vi "Blend.vi"(7 "Source Name in":string, 8 "error in (no error)":errorcluster, 9 "Source Enqueuer":refnum<class "Message Enqueuer.lvclass">, 10 "Sample to Blend in":refnum<class "Sample.lvclass">, 11 "Preparation Line in":refnum<class "Preparation Line.lvclass">) -> (0 "error out":errorcluster, 2 "Source Name":string, 3 "Preparation Line out":refnum<class "Preparation Line.lvclass">)   [LabVIEW 2015, in "cRIO-Carbondioxide.lvlib" / "CO2-Actor.lvlib" / "Preparation Line.lvclass"]
uses:
  Preparation Line.lvclass
  subs/Sample/Sample.lvclass
  <vilib>/ActorFramework/Message Enqueuer/Message Enqueuer.lvclass
  Valve/Valve.lvclass
  Preparation Line.lvclass/Preparation Line.ctl
  CO2 Actor Messages/Ping Msg/Ping Msg.lvclass/Ping Msg.ctl
  <vilib>/ActorFramework/Message Enqueuer/Message Enqueuer.lvclass/Message Enqueuer.ctl
  <vilib>/ActorFramework/Message Enqueuer/Enqueue.vi
  <vilib>/ActorFramework/Message Priority Queue/Priority Enqueue.vi
  CO2 Actor/CO2 Actor.lvclass
  CO2 Actor Messages/Ping Msg/Ping Msg.lvclass
  <vilib>/ActorFramework/Actor/Actor.lvclass
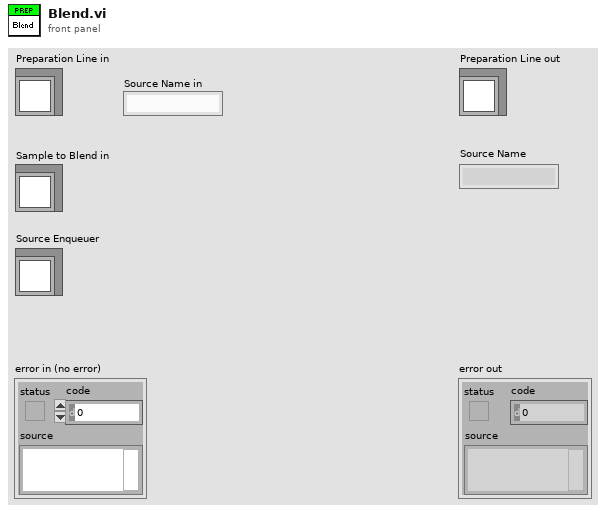
[diagram p1: front panel]
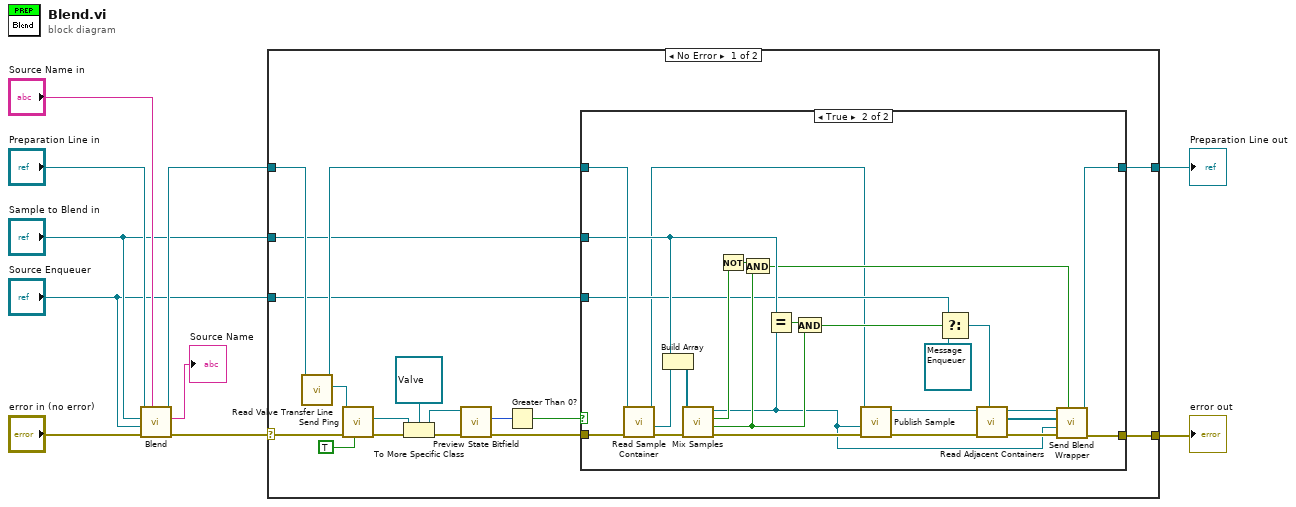
[diagram p0: block diagram]
diagram:
  n1 = call-parent "Blend.vi"("Source Name in"="Source Name in", "error in (no error)"="error in (no error)", "Source Enqueuer"="Source Enqueuer", "Sample to Blend in"="Sample to Blend in", "CO2 Actor in"="Preparation Line in") -> ("error out"=w4:errorcluster, "Source Name"=→"Source Name":string, "CO2 Actor out"=w6:refnum<class "Preparation Line.lvclass">)  [unwired: 4 in]
  n2 = case shown="No Error" w4 {
    selector: w4 -> [w26 w56]
    tunnel: w6 -> [w27 w55]
    tunnel: [w14 w55] -> w5
    tunnel: "Sample to Blend in" -> [w16 _]
    tunnel: "Source Enqueuer" -> [w15 _]
    tunnel: [w13 w56] -> w1
    frame No Error {
      n3 = call "Read Valve Transfer Line.vi"("Preparation Line in"=w27) -> ("Actor Framework:Message Enqueuer"=w25:refnum<class "Message Enqueuer.lvclass">, "Preparation Line out"=w17:refnum<class "Preparation Line.lvclass">)  [unwired: 9 in]
      n4 = call "Send Ping.vi"("Return Self (F)"=TRUE, "error in (no error)"=w26, "Message Enqueuer"=w25) -> ("error out"=w24:errorcluster, "Actor out"=w23:refnum<class "Actor.lvclass">)  [unwired: 5 in, 2 out]
      n5 = To More Specific Class(target class=refnum<class "Valve.lvclass"> refnum ("Valve.lvclass"), reference=w23, error in=w24) -> (specific class reference=w19:refnum<class "Valve.lvclass">, error out=w21:errorcluster)
      n6 = call "Preview State Bitfield.vi"("error in (no error)"=w21, "Valve in"=w19) -> ("error out"=w20:errorcluster, "State Bitfield"=w18:u16)  [unwired: 7 in, 1 out]
      n7 = Greater Than 0?(x=w18) -> (x > 0?=w12:bool)
      n8 = case shown="True" w12 {
        tunnel: w20 -> [w28 w54]
        tunnel: w17 -> [w29 w50]
        tunnel: w16 -> [_ w48]
        tunnel: w15 -> [_ w41]
        tunnel: [w29 w32] -> w14
        tunnel: [w28 w31] -> w13
        frame False {
        }
        frame True {
          n9 = call "Read Sample Container.vi"("error in (no error)"=w54, "Preparation Line in"=w50) -> ("error out"=w53:errorcluster, "Sample"=w52:refnum<class "Sample.lvclass">, "Preparation Line out"=w33:refnum<class "Preparation Line.lvclass">)  [unwired: 6 in, 1 out]
          n10 = Build Array(w48, w52) -> (w51:refnum<class "Sample.lvclass">[])
          n11 = call "Mix Samples.vi"("error in (no error)"=w53, "Samples In"=w51) -> ("error out"=w49:errorcluster, "is clean?"=w43:bool, "Empty Samples present?"=w46:bool, "Sample out"=w30:refnum<class "Sample.lvclass">)  [unwired: 6 in]
          n12 = Not(x=w46) -> (.not. x?=w47:bool)
          n13 = And(x=w47, y=w43) -> (x .and. y?=w45:bool)
          n14 = Equal?(x=w48, y=w30) -> (x = y?=w44:bool)
          n15 = And(x=w44, y=w43) -> (x .and. y?=w42:bool)
          n16 = call "Publish Sample.vi"("error in (no error)"=w49, "Sample"=w30, "Preparation Line in"=w33) -> ("error out"=w38:errorcluster, "Preparation Line out"=w37:refnum<class "Preparation Line.lvclass">)  [unwired: 7 in]
          n17 = Select(t=w41, s=w42, f=refnum<class "Message Enqueuer.lvclass"> refnum) -> (s? t:f=w39:refnum<class "Message Enqueuer.lvclass">)
          n18 = call "Read Adjacent Containers.vi"("Exclude Source"=w39, "error in (no error)"=w38, "Preparation Line in"=w37) -> ("error out"=w34:errorcluster, "Adjacent Containers"=w36:refnum<class "Message Enqueuer.lvclass">[], "Preparation Line out"=w35:refnum<class "Preparation Line.lvclass">)  [unwired: 6 in]
          n19 = call-dynamic "Send Blend Wrapper.vi"("Include Source EnQr (T)"=w45, "error in (no error)"=w34, "Sample to Blend"=w30, "Send to"=w36, "CO2 Actor in"=w35) -> ("error out"=w31:errorcluster, "CO2 Actor out"=w32:refnum<class "Preparation Line.lvclass">)  [unwired: 5 in]
        }
      }
    }
    frame Error {
    }
  }
  "error out" <- w1
  "Preparation Line out" <- w5
